vi "UHR-Fleezers Control (fpga) - 9.3.vi"() -> ()   [LabVIEW 2009]
doc: "UHR-Fleezers Instrument Control Code (fpga)"
uses:
  <vilib>/Platform/TimedLoop/XDataNode/XDataNode.xnode
  <vilib>/Platform/TimedLoop/XDataNode/loadlvalarms.vi
  <vilib>/Platform/TimedLoop/XDataNode/timing_clust.ctl
  <vilib>/Platform/TimedLoop/XDataNode/nitl_modes.ctl
  <vilib>/Platform/TimedLoop/XDataNode/wakeup.ctl
  <vilib>/eio/EIONode/EIONode.xnode
  <vilib>/rvi/eio/nirviEIOImplementation/nirviEIOImplementation.xnode
  <vilib>/rvi/eio/common/nirviEmuTemplateMethod_noerrors.vi
  <vilib>/rvi/eio/common/nirviEmuClasses.ctl
  <vilib>/eio/EIOMethodNode/EIOMethodNode.xnode
  <vilib>/rvi/eio/nirviEIOMethodImplementation/nirviEIOMethodImplementation.xnode
  <vilib>/rvi/DataTransferAndStorage/Container/XNode/niFpgaContainer.xnode
  <vilib>/rvi/interface/RandomDataEmulation/niFpgaRandomDataHandleErrors.vi
  <vilib>/rvi/interface/RandomDataEmulation/nirviRandomDataFPGAFIFO.vi
  <vilib>/rvi/DataTransferAndStorage/Container/Common/niFpgaContainerMethod.ctl
  <vilib>/rvi/DataTransferAndStorage/Container/Common/niFpgaTransferTypeControl.ctl
  <vilib>/Platform/TimedLoop/XDataNode/XDNodeRunTimeDep.lvlib
panel:
  in  "Tab Control":T1(tab)=enum."APD Counting"
  in  "AI Averages":u16=1 min=1 step=1
  in  "AI1 Sets to FIFO":T2={"Set 1"=TRUE, "Set 2"=TRUE, "Set 3"=FALSE}
  in  "N of AI1 Int Acq Sets":i16=2 min=1 max=3 step=1
  out "Number of AI channels":i16
  out "AI Late Counter":u32
  in  "ai count":u32=400
  out "AI late?":bool
  in  "+ phase":bool
  in  "Phase count adjustment":i16
  out "Relative phase":i16
  in  "DMA buffer timeout":i32
  in  "AI to FIFO":bool
  in  "Tab Control 2":T3(tab)
  in  "Swap F1 and F2":bool
  in  "Freq or Amp switch first":bool=TRUE
  in  "Cont. Scan":bool
  in  "Abort scan":bool
  in  "Cycles per step":u64
  in  "Scan BD":bool
  in  "Number of scans":u16
  in  "Scan steps":u64
  in  "Scan freq.  increment":i64
  out "Scanning":bool
  in  "Start scan":bool
  in  "OSK Bd 1":bool
  in  "Reset Bd 1":bool
  in  "RD":bool
  in  "PMODE":bool
  in  "OSK Bd 2":bool
  in  "Reset Bd 2":bool
  in  "Direct RF Box \nCommunication":bool
  in  "Data BD 2":u8 format="%08b"
  in  "Data BD 1":u8 format="%08b"
  in  "Address":u8 format="%02x"
  in  "Update Data":bool
  in  "FPGA Controls\n RF Box":bool
  in  "Number Interlace Cycles":u8=2 min=1 max=3
  in  "Interlace Off Parameters":u8=1 min=1 max=3
  in  "Interlace ON/OFF":bool
  out "DIO Relative phase":i16
  in  "Phase count adjustment (DIO)":i16
  in  "+ phase (DIO)":bool
  out "DIO Late Counter":u32
  out "DIO Late?":bool
  in  "DIO count 1 (ticks)":u32=400
  in  "DIO count 2 (ticks)":u32=400
  in  "DIO count 3 (ticks)":u32=400
  out "AI2 Y Sum Set 2":i16
  out "AI2 Y Sum Set 1":i16
  in  "FB Gains Set 1":T4={"proportional gain (Kc)"=10, "integral gain (Kc*Ts/Ti)"=5, "derivative gain (Kc*Td/Ts)"=0}
  in  "FB Setpoint Set 1":i16 min=0 step=1
  in  "FB Reset Set 1":bool
  in  "FB On/Off Set 1":bool
  in  "FB Reset Set 2":bool
  in  "FB On/Off Set 2":bool
  in  "FB Setpoint Set 2":i16 min=0 step=1
  in  "FB Gains Set 2":T4={"proportional gain (Kc)"=10, "integral gain (Kc*Ts/Ti)"=5, "derivative gain (Kc*Td/Ts)"=0}
  in  "FB output range 2":cluster{"output high":i16, "output low":i16}={"output high"=3000, "output low"=0}
  in  "FB output range 1":cluster{"output high":i16, "output low":i16}={"output high"=3000, "output low"=0}
  out "Scan I":u64
  in  "Amp switch delay":u16=5
  in  "Freq switch delay":u16
  in  "BD 2 Amplitude 1":u16
  in  "BD 1 Amplitude 1":u16
  in  "BD 2 Frequency 1":u64
  in  "BD 1 Frequency 1":u64
  in  "BD 2 Amplitude 2":u16
  in  "BD 1 Amplitude 2":u16
  in  "BD 2 Frequency 2":u64
  in  "BD 1 Frequency 2":u64
  in  "BD 2 Amplitude 3":u16
  in  "BD 1 Amplitude 3":u16
  in  "BD 2 Frequency 3":u64
  in  "BD 1 Frequency 3":u64
  out "Numeric":i32
  out "AO2 2":i16
  out "AO1 2":i16
  in  "1D or 2D Scan?":bool
  in  "Abort scan (MCL)":bool
  in  "MCL Scan Axis":bool
  in  "Cont. Scan (MCL)":bool
  out "Scan I (MCL)":u64
  in  "Number of scans (MCL)":u16
  out "Scanning MCL":bool
  in  "Scan steps (MCL)":u64
  in  "Cycles per step (MCL)":u64
  in  "Scan freq.  increment (MCL)":i16
  in  "Start scan (MCL)":bool
  in  "AO2":i16
  in  "AO1":i16
  out "MCL Late Counter":u32
  out "MCL Late?":bool
  in  "MCL count":u32=800
  out "MCL Relative Phase":i16
  in  "Phase count adjustment (MCL)":i16
  in  "+ phase (MCL)":bool
  in  "APD2 Trigger on Edge?":bool=TRUE
  in  "APD1 Trigger on Edge?":bool=TRUE
  in  "APD Gate Operating Mode":u8 max=2 step=1
  in  "Invert APD Gate":bool
  in  "APD Gate OFF Count":u32=100
  in  "APD Gate ON Count":u32=300
  out "APD Gate Late Counter":u32
  out "APD Gate Late?":bool
  out "APD Gate Relative Phase":i16
  in  "Phase count adjustment (APD Gate)":i16
  in  "+ phase (APD Gate)":bool
  out "APD 2 Counts 0":u32
  out "APD 2 Counts 1":u32
  out "APD 1 Counts 0":u32
  out "APD 1 Counts 1":u32
  out "APD out state":bool
  in  "APD 2 AO offset":i16
  in  "APD 1 AO offset":i16
  in  "APD 2 AO scale factor":i16=1
  in  "APD 1 AO scale factor":i16=1
  in  "APD to FIFO":bool
  in  "APD Acq Rate Count":u32=20000000
  out "APD Acq Late Counter":u32
  out "APD Acq Late?":bool
  out "APD Acq Relative Phase":i16
  in  "Phase Count Adjustment (APD Acq)":i16
  in  "+ phase (APD Acq)":bool
  in  "Green Filter Flipper":bool
  out "Green FB Signals":T5
  in  "Green FB Count":u32=1200
  out "Green Late Counter":u32
  out "Green FB Late?":bool
  out "Green FB Relative Phase":i16
  in  "Phase count adjustment (Green FB)":i16=10
  in  "+ phase (Green FB)":bool
  out "Green FB Sum":i16
  in  "Green int current ON count adj":u32=150
  in  "Current Out":u16=30000
  in  "Green FB On/Off":bool
  in  "Green FB Setpoint":i16=250 min=0 step=1
  in  "Green FB Gains":T4={"proportional gain (Kc)"=10, "integral gain (Kc*Ts/Ti)"=5, "derivative gain (Kc*Td/Ts)"=0}
  in  "Green FB Reset":bool
  in  "Operating Mode 2":u8=2 max=2 step=1
  in  "Invert GI 2":bool
  in  "Green interlace OFF count 2":u32=900
  in  "Green interlace ON count 2":u32=300
  out "GI Late Counter 2":u32
  out "GI Late? 2":bool
  out "GI Relative phase 2":i16
  in  "Phase count adjustment (GI) 2":i16=20
  in  "+ phase (GI) 2":bool
  in  "Green interlace OFF count":u32=100
  out "GI Relative phase":i16
  in  "Phase count adjustment (GI)":i16
  in  "+ phase (GI)":bool
  out "GI Late?":bool
  in  "Green interlace ON count":u32=300
  out "GI Late Counter":u32
  in  "Invert GI":bool
  in  "Operating Mode":u8 max=2 step=1
  in  "Connector0/DIO9":bool
  in  "Connector1/DIO32":bool
  in  "Connector1/DIO33":bool
  in  "Connector1/DIO34":bool
  in  "Chassis2/Mod4/AO1":u16
  in  "Extra DO Counts":u32=40000
  # "Only one of these can be on\nat a time:"
  # "Raster Scan AOD"
  # "1 (X)"
  # "2 (Y)"
  # "IR Intensity Feedback (RF BD 1)"
  # "AO1 (Y)"
  # "2D"
  # "1D"
  # "AO2 (X)"
  # "APD AO for aligning"
  # "Detection Loop"
  # "Green fluorescent laser digital gate interlacing loop"
  # "0 Forced ON\n1 Forced OFF\n2 Interlacing"
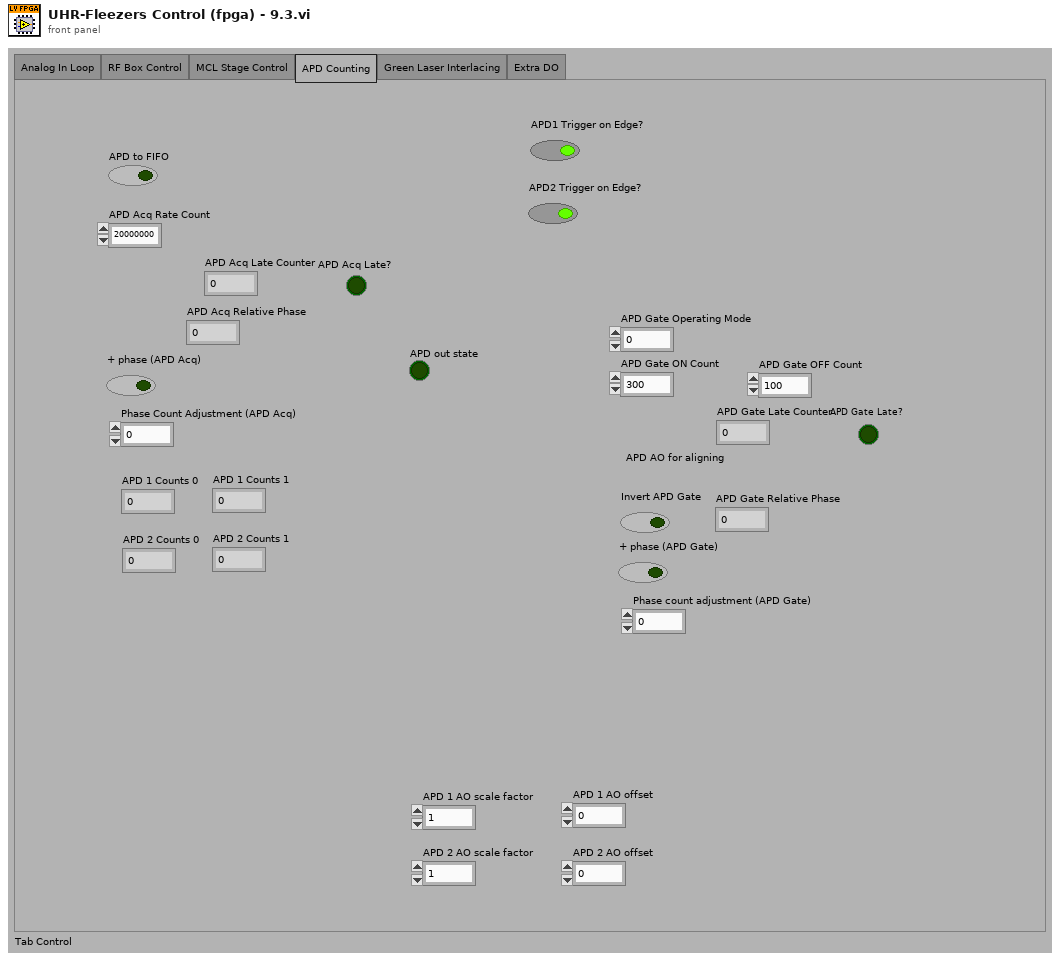
[diagram p1: front panel]
types:
  T1 = enum32{"Analog In Loop", "RF Box Control", "MCL Stage Control", "APD Counting", "Green Laser Interlacing", "Extra DO"}
  T2 = cluster{"Set 1":bool, "Set 2":bool, "Set 3":bool}
  T3 = enum32{"Controls", "Interlacing Frequency and Amplitude Values"}
  T4 = cluster{"proportional gain (Kc)":i16, "integral gain (Kc*Ts/Ti)":i16, "derivative gain (Kc*Td/Ts)":i16}
  T5 = cluster{"Green FB Ch 0":i16, "Green FB Ch 1":i16, "Green FB Ch 2":i16}
  T6 = typedef "nirviEmuClasses.ctl" = enum16{"IO Read", "IO Write", "Method", "Property Read", "Property Write"}
  T7 = typedef "XDNodeRunTimeDep.lvlib/timing_clust.ctl" = cluster{"Expected End [f-1]":u64, "Actual End [f-1]":u64, "Finished Late? [f-1]":bool, "Expected End [i-1]":u64, "Actual End [i-1]":u64, "Finished Late? [i-1]":bool, "Expected Start [i]":u64, "Actual Start [i]":u64, "Expected Start [f]":u64, "Actual Start [f]":u64, "Source Name":string, "Structure Name":string, "Period":i64, "Deadline":i64, "Offset":i64, "Start":i64, "Priority":i32, "Timeout":i32, "Mode":T8, "Wakeup Reason":T9, "Error":errorcluster, "Source Type":string, "Secondary Source Type":string, "Global End Time":u64, "Global Start Time":u64, "Frame Duration":u64, "Iteration Duration":u64, "Assigned CPU":i32, "I/O Scan Engine Mode":u32}
  T8 = typedef "XDNodeRunTimeDep.lvlib/nitl_modes.ctl" = enum32{"No Change", "Process missed periods, maintain original phase", "Discard missed periods, maintain original phase", "Process missed periods, ignore original phase", "Discard missed periods, ignore original phase"}
  T9 = typedef "XDNodeRunTimeDep.lvlib/wakeup.ctl" = enum32{"Normal", "Aborted", "Asynchronous wakeup", "Timing source error", "Timed loop error", "Timeout"}
  T10 = typedef "niFpgaContainerMethod.ctl" = enum16{"Write", "Read", "Clear", "Get Number of Elements to Write", "Get Number of Elements to Read", "Enable", "Disable", "Flush and Disable", "Get Stream State"}
  T11 = typedef "niFpgaTransferTypeControl.ctl" = enum16{"Target-Scoped", "Host to Target - DMA", "Target to Host - DMA", "Peer to Peer Reader", "Peer to Peer Writer", "Bidirectional"}
  T12 = cluster{"Chassis2/Mod1/AI0":i16, "Chassis2/Mod1/AI1":i16, "Chassis2/Mod1/AI2":i16}
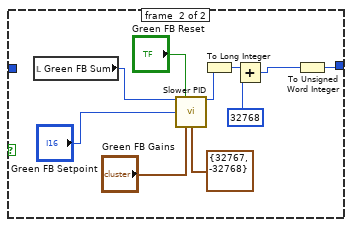
[diagram p2: hidden frame]
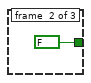
[diagram p3: hidden frame]
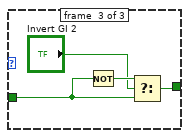
[diagram p4: hidden frame]
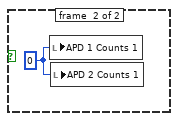
[diagram p5: hidden frame]
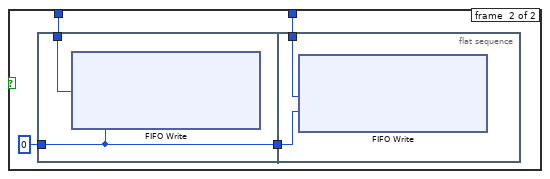
[diagram p6: hidden frame]
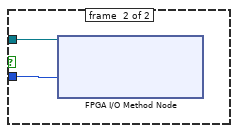
[diagram p7: hidden frame]
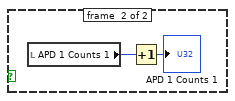
[diagram p8: hidden frame]
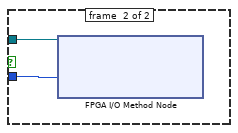
[diagram p9: hidden frame]
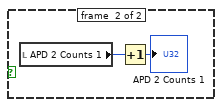
[diagram p10: hidden frame]
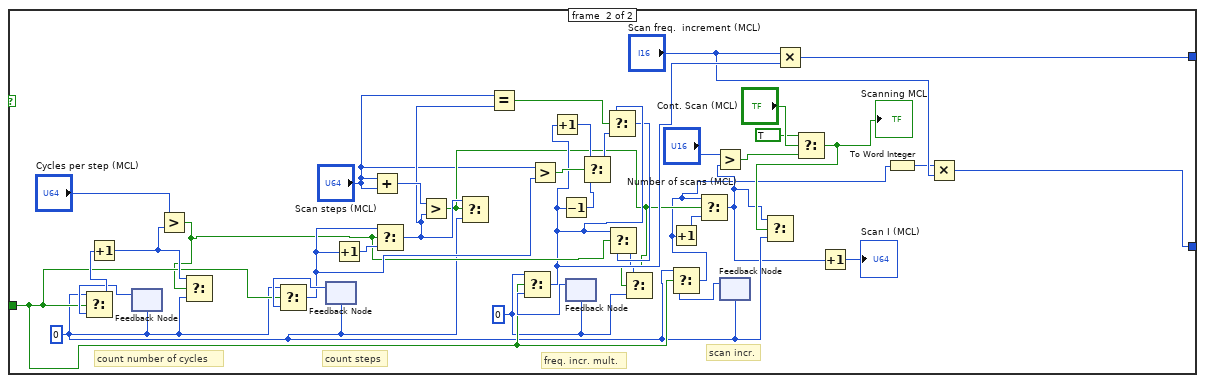
[diagram p11: hidden frame]
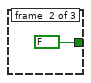
[diagram p12: hidden frame]
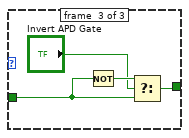
[diagram p13: hidden frame]
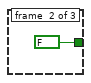
[diagram p14: hidden frame]
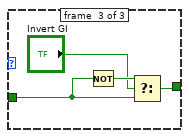
[diagram p15: hidden frame]
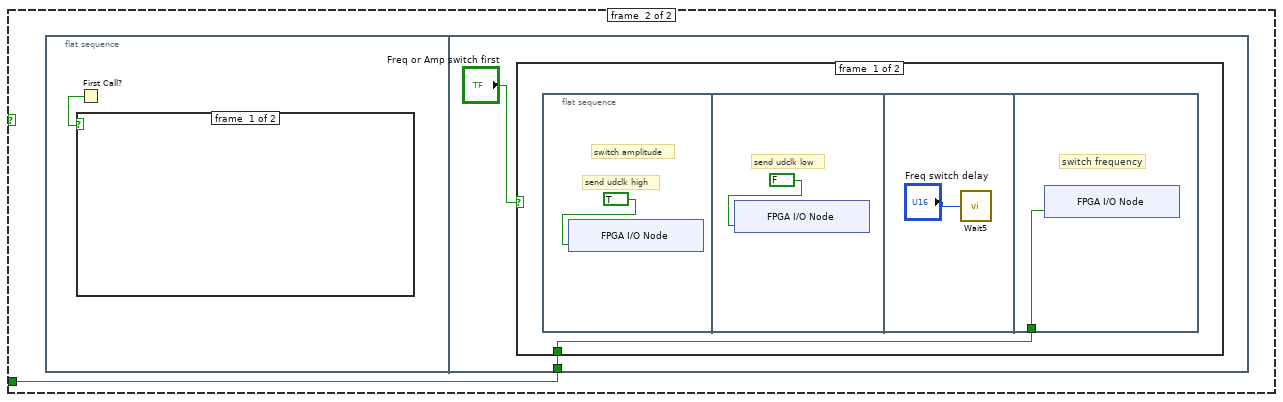
[diagram p16: hidden frame]
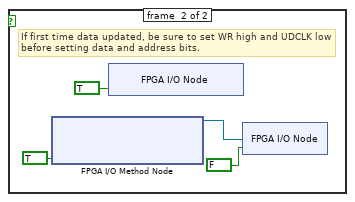
[diagram p17: hidden frame]
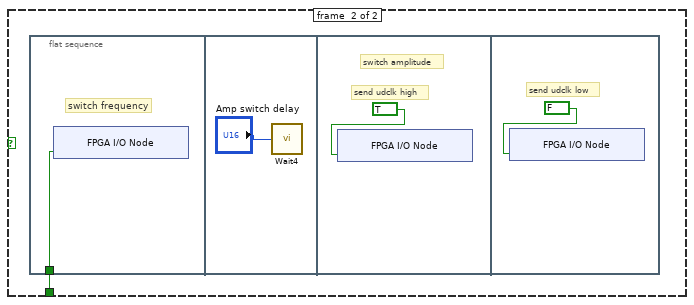
[diagram p18: hidden frame]
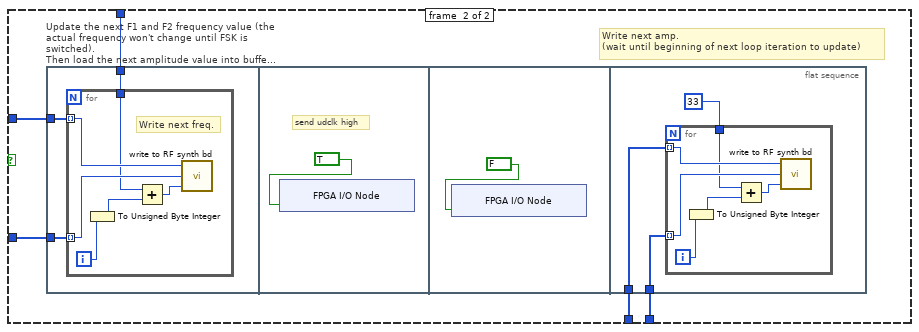
[diagram p19: hidden frame]
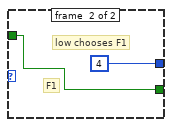
[diagram p20: hidden frame]
diagram:
  # "timing array current index"
  # "timing array"
  # "timing counter (phase adjusted here)"
  # "late counter"
  n1 = flat-sequence "FPGA initialization to do before running any of the loops" {
    tunnel: [u32 0 ("DIO count 3 (ticks)")] -> w1
    tunnel: [w10] -> _
    frame #0 {
      # "This is a kludge to let host programs know how many channels of data are in the DMA stream.  Set by hand."
      # "Start up expansion chassis early\nto avoid delays later"
      # "This pin controls udclk on the RF boards.\nWhen initially configuring the boards, this pin needs to be\nconfigured as a high impedance input.  Later it will be switched\nto an output."
      # "Initial setting of DIO data and \naddress to low (before reset).  \nThis needs to happen before the other\ncontrol method loops execute."
      n2 = xnode "FPGA I/O Node"("Chassis2/Mod4/AO0"=u16 0) -> ("Chassis2/Mod1/AI0"=w10:i16)  [unwired: 2 in, 2 out]
      n3 = xnode "FPGA I/O Method Node"("Enable"=FALSE) -> ()  [unwired: 1 in, 1 out]
      n4 = xnode "FPGA I/O Node"("Connector1/DIO0"=FALSE, "Connector1/DIO1"=FALSE, "Connector1/DIO2"=FALSE, "Connector1/DIO3"=FALSE, "Connector1/DIO4"=FALSE, "Connector1/DIO5"=FALSE, "Connector1/DIO6"=FALSE, "Connector1/DIO7"=FALSE, "Connector1/DIO8"=FALSE, "Connector1/DIO9"=FALSE, "Connector1/DIO10"=FALSE, "Connector1/DIO11"=FALSE, "Connector1/DIO12"=FALSE, "Connector1/DIO13"=FALSE, "Connector1/DIO15"=FALSE, "Connector1/DIO20"=FALSE, "Connector1/DIO21"=FALSE, "Connector1/DIO22"=FALSE, "Connector1/DIO23"=FALSE, "Connector1/DIO24"=FALSE, "Connector1/DIO25"=FALSE, "Connector1/DIO26"=FALSE, "Connector1/DIO27"=FALSE, "Connector1/DIO14"=FALSE) -> ()  [unwired: 24 in, 24 out]
      "Number of AI channels" <- i16 12 ("Number of AI channels")
    }
  }
  n5 = local read "AO1"() -> (w5:i16)
  n6 = local read "AO2"() -> (w4:i16)
  n7 = node-c288() -> (w3:T7)  [unwired: 1 in]
  n8 = while "APD 1 Counter" {
    tunnel: w1 -> [_]
    stop <- FALSE stop-if-true
    n9 = flat-sequence {
      frame #0 {
        n10 = case shown="False" "APD1 Trigger on Edge?" {
          tunnel: refnum<k21> "Connector0/DIO0" ("APD 1 DO") -> [w398 w423]
          tunnel: -1 ("Timeout") -> [w397 w422]
          frame #0 {
            n11 = xnode "FPGA I/O Method Node"("FPGA I/O In"=w398, "Timeout"=w397) -> ()  [unwired: 2 out]
          }
          frame #1 {
            n12 = xnode "FPGA I/O Method Node"("FPGA I/O In"=w423, "Timeout"=w422) -> ()  [unwired: 2 out]
          }
        }
      }
      frame #1 {
        n13 = local read "APD out state"() -> (w447:bool)
        n14 = case shown="False" w447 {
          frame #0 {
            n15 = local read "APD 1 Counts 0"() -> (w449:u32)
            n16 = Increment(x=w449) -> (x+1=→"APD 1 Counts 0":u32)
          }
          frame #1 {
            n17 = local read "APD 1 Counts 1"() -> (w451:u32)
            n18 = Increment(x=w451) -> (x+1=→"APD 1 Counts 1":u32)
          }
        }
      }
    }
  }
  n19 = while "APD 2 Counter" {
    tunnel: w1 -> [_]
    stop <- FALSE stop-if-true
    n20 = flat-sequence {
      frame #0 {
        n21 = case shown="False" "APD2 Trigger on Edge?" {
          tunnel: refnum<k21> "Connector0/DIO1" ("APD 2 DO") -> [w457 w482]
          tunnel: -1 ("Timeout") -> [w456 w481]
          frame #0 {
            n22 = xnode "FPGA I/O Method Node"("FPGA I/O In"=w457, "Timeout"=w456) -> ()  [unwired: 2 out]
          }
          frame #1 {
            n23 = xnode "FPGA I/O Method Node"("FPGA I/O In"=w482, "Timeout"=w481) -> ()  [unwired: 2 out]
          }
        }
      }
      frame #1 {
        n24 = local read "APD out state"() -> (w506:bool)
        n25 = case shown="False" w506 {
          frame #0 {
            n26 = local read "APD 2 Counts 0"() -> (w508:u32)
            n27 = Increment(x=w508) -> (x+1=→"APD 2 Counts 0":u32)
          }
          frame #1 {
            n28 = local read "APD 2 Counts 1"() -> (w510:u32)
            n29 = Increment(x=w510) -> (x+1=→"APD 2 Counts 1":u32)
          }
        }
      }
    }
  }
  n30 = while "DAQ AI set 1" {
    shift-right: [w511] -> _
    shift-left: w1 -> [w516]
    stop <- FALSE stop-if-true
    n31 = flat-sequence {
      tunnel: w516 -> [w526]
      tunnel: [w527] -> w514
      tunnel: [w526] -> w513
      tunnel: [w537] -> w524
      tunnel: [w536] -> w523
      tunnel: [w535] -> w522
      tunnel: [w534] -> w521
      tunnel: [w533] -> w520
      tunnel: [w532] -> w519
      tunnel: [w531] -> w518
      tunnel: [w530] -> w517
      tunnel: [w529] -> w515
      tunnel: w514 -> [w529]
      tunnel: w513 -> [w528]
      tunnel: [w528] -> w512
      tunnel: [w714] -> w511
      tunnel: w524 -> [w752]
      tunnel: w523 -> [w751]
      tunnel: w522 -> [w735]
      tunnel: w521 -> [w750]
      tunnel: w520 -> [w739]
      tunnel: w519 -> [w738]
      tunnel: w518 -> [w737]
      tunnel: w517 -> [w736]
      tunnel: w515 -> [w731]
      tunnel: w512 -> [w728]
      frame #0 {
        n32 = call "Loop Timer3"("Count(Ticks)"=w526) -> ("Tick Count(Ticks)"=w527:u32)
      }
      frame #1 {
        n33 = xnode "FPGA I/O Node"("Connector1/DIO31"=TRUE ("Connector1/DIO33")) -> ("Connector0/AI0"=w537:i16, "Connector0/AI1"=w536:i16, "Connector0/AI2"=w535:i16, "Connector0/AI3"=w534:i16, "Connector0/AI4"=w533:i16, "Connector0/AI5"=w532:i16, "Connector0/AI6"=w531:i16, "Connector0/AI7"=w530:i16)  [unwired: 9 in, 9 out]
      }
      frame #2 {
        # "Adjust phase after data acquired if button pressed"
        n34 = feedback #1(i16 1) -> (w743:i16)
        n35 = Increment(x=w743) -> (x+1=w749:i16)
        n36 = Greater?(x=w749, y="N of AI1 Int Acq Sets") -> (0:w746:bool)
        n37 = Select(t=i16 1, s=w746, f=w749) -> (s? t:f=w748:i16)
        n38 = feedback #2(FALSE ("AI to FIFO")) -> (w733:bool)
        n39 = case shown="1, Default" w743 {
          tunnel: w735 -> [w755 w759 _]
          tunnel: "AI1 Sets to FIFO" -> [w757 w761 w764]
          tunnel: [w756 w760 w763] -> w740
          tunnel: ["AI to FIFO" w758 w762] -> w732
          tunnel: w733 -> [_ w758 w762]
          frame #0 {
            n40 = Unbundle By Name(w757) -> ("Set 1"=w756:bool)
            "AI2 Y Sum Set 1" <- w755
          }
          frame #1 {
            n41 = Unbundle By Name(w761) -> ("Set 2"=w760:bool)
            "AI2 Y Sum Set 2" <- w759
          }
          frame #2 {
            n42 = Unbundle By Name(w764) -> ("Set 3"=w763:bool)
          }
        }
        n43 = And(x=w740, y=w732) -> (x .and. y?=w742:bool)
        n44 = case shown="True" w742 {
          tunnel: w752 -> [_ w769]
          tunnel: w751 -> [_ w770]
          tunnel: w735 -> [_ w771]
          tunnel: w750 -> [_ w772]
          tunnel: w739 -> [_ w776]
          tunnel: w738 -> [_ w775]
          tunnel: w737 -> [_ w774]
          tunnel: w736 -> [_ w773]
          frame #0 {
          }
          frame #1 {
            n45 = Greater?(x="AI Averages", y=u16 1) -> (0:w767:bool)
            n46 = case shown="True" w767 {
              tunnel: w776 -> [w787 w844]
              tunnel: w775 -> [w786 w843]
              tunnel: w774 -> [w785 w842]
              tunnel: w773 -> [w784 w841]
              tunnel: w772 -> [w783 w840]
              tunnel: w771 -> [w788 w839]
              tunnel: w770 -> [w789 w838]
              tunnel: w769 -> [w790 w837]
              tunnel: "AI Averages" -> [_ w824]
              tunnel: "DMA buffer timeout" -> [w778 w821]
              frame #0 {
                n47 = Join Numbers(hi=w790, lo=w789) -> ((hi.lo)=w782:u32)
                n48 = Join Numbers(hi=w788, lo=w783) -> ((hi.lo)=w781:u32)
                n49 = Join Numbers(hi=w787, lo=w786) -> ((hi.lo)=w780:u32)
                n50 = Join Numbers(hi=w785, lo=w784) -> ((hi.lo)=w779:u32)
                n51 = Build Array(w782, w781, w780, w779) -> (w777:u32[])
                n52 = for {
                  tunnel: w777 -> [w792] mode=indexing
                  tunnel: w778 -> [w793]
                  n53 = To Unsigned Long Integer(number=w792) -> (unsigned 32bit integer=w791:u32)
                  n54 = xnode ("FIFO Write")("Element"=w791, "Timeout"=w793) -> ()  [unwired: 1 in, 2 out]
                }
              }
              frame #1 {
                w828 = u16 0
                n55 = To Long Integer(number=w837) -> (32bit integer=w830:i32)
                n56 = To Long Integer(number=w838) -> (32bit integer=w847:i32)
                n57 = To Long Integer(number=w839) -> (32bit integer=w846:i32)
                n58 = To Long Integer(number=w840) -> (32bit integer=w845:i32)
                n59 = To Long Integer(number=w844) -> (32bit integer=w836:i32)
                n60 = To Long Integer(number=w843) -> (32bit integer=w835:i32)
                n61 = To Long Integer(number=w842) -> (32bit integer=w834:i32)
                n62 = To Long Integer(number=w841) -> (32bit integer=w833:i32)
                n63 = Build Array(w830, w847, w846, w845, w836, w835, w834, w833) -> (w819:i32[])
                n64 = feedback #3(w819) -> (w832:i32[])
                n65 = Add(x=w819, y=w832) -> (x+y=w831:i32[])
                n66 = feedback #4(w828) -> (w826:u16)
                n67 = Increment(x=w826) -> (x+1=w823:u16)
                n68 = Equal?(x=w823, y=u16 1) -> (x = y?=w822:bool)
                n69 = Select(t=w819, s=w822, f=w831) -> (s? t:f=w820:i32[])
                n70 = Greater Or Equal?(x=w823, y=w824) -> (x >= y?=w825:bool)
                n71 = Select(t=w828, s=w825, f=w823) -> (s? t:f=w827:u16)
                n72 = case shown="True" w825 {
                  tunnel: w820 -> [_ w849]
                  tunnel: w821 -> [_ w848]
                  frame #0 {
                  }
                  frame #1 {
                    n73 = for {
                      tunnel: w849 -> [w851] mode=indexing
                      tunnel: w848 -> [w852]
                      n74 = To Unsigned Long Integer(number=w851) -> (unsigned 32bit integer=w850:u32)
                      n75 = xnode ("FIFO Write")("Element"=w850, "Timeout"=w852) -> ()  [unwired: 1 in, 2 out]
                    }
                  }
                }
              }
            }
          }
        }
        n76 = feedback #5(w731) -> (w730:u32)
        n77 = Subtract(x=w731, y=w730) -> (x-y=w729:u32)
        n78 = Subtract(x=w729, y=w728) -> (x-y=w725:u32)
        n79 = Subtract(x="ai count", y=w725) -> (x-y=w715:u32)
        n80 = Greater?(x=w725, y=u32 0) -> (0:w723:bool)
        "AI late?" <- w723
        n81 = feedback #6(u32 0) -> (w721:u32)
        n82 = Increment(x=w721) -> (x+1=w720:u32)
        n83 = Select(t=w720, s=w723, f=w721) -> (s? t:f=w722:u32)
        "AI Late Counter" <- w722
        n84 = xnode "I/O Node"("Connector1/DIO31"=FALSE ("Connector1/DIO34")) -> ()  [unwired: 1 in, 1 out]
        n85 = Boolean To (0,1)(Boolean="+ phase") -> (0, 1=w717:i16)
        n86 = Multiply(x=w717, y="Phase count adjustment") -> (x*y=w711:i16)
        n87 = feedback #7(i16 0) -> (w713:i16)
        n88 = Add(x=w715, y=w711) -> (x+y=w714:u32)
        n89 = Subtract(x=w713, y=w711) -> (x-y=w712:i16)
        "Relative phase" <- w712
      }
    }
  }
  n90 = while "RF box board DIO control: parallel communication" {
    shift-right: [w897] -> _
    shift-left: w1 -> [w896]
    shift-right: [w895] -> _
    shift-left: FALSE ("Swap F1 and F2") -> [w894]
    stop <- FALSE stop-if-true
    n91 = flat-sequence {
      tunnel: w894 -> [w901]
      tunnel: w896 -> [w899]
      tunnel: [w901] -> w893
      tunnel: [w900] -> w892
      tunnel: [w899] -> w891
      tunnel: [w907] -> w897
      tunnel: [w906] -> w895
      tunnel: w893 -> [w905]
      tunnel: w892 -> [w903]
      tunnel: w891 -> [w902]
      frame #0 {
        n92 = call "Loop Timer"("Count(Ticks)"=w899) -> ("Tick Count(Ticks)"=w900:u32)
      }
      frame #1 {
        n93 = flat-sequence {
          tunnel: ["FPGA Controls\n RF Box"] -> w904
          tunnel: w905 -> [w908]
          tunnel: [w1057] -> w907
          tunnel: [w1077] -> w906
          tunnel: w904 -> [w1076]
          tunnel: w903 -> [w1070]
          tunnel: w902 -> [w1067]
          frame #0 {
            n94 = case shown="True" "FPGA Controls\n RF Box" {
              tunnel: w908 -> [_ w910]
              frame #0 {
              }
              frame #1 {
                n95 = flat-sequence {
                  tunnel: w910 -> [w955]
                  frame #0 {
                    n96 = First Call?() -> (First Call?: T/F=w911:bool)
                    n97 = case shown="True" w911 {
                      frame #0 {
                      }
                      frame #1 {
                        # "If first time data updated, be sure to set WR high and UDCLK low\nbefore setting data and address bits."
                        n98 = xnode "FPGA I/O Method Node"("Enable"=TRUE) -> ("FPGA I/O Out"=w913:refnum<k21>)  [unwired: 1 in]
                        n99 = xnode "FPGA I/O Node"("Connector1/DIO15"=TRUE) -> ()  [unwired: 1 in, 1 out]
                        n100 = xnode "FPGA I/O Node"("I/O Item"=FALSE ("Connector1/DIO30"), "FPGA I/O In"=w913) -> ()  [unwired: 1 out]
                      }
                    }
                  }
                  frame #1 {
                    n101 = case shown="True" "Freq or Amp switch first" {
                      tunnel: w955 -> [w957 w1001]
                      frame #0 {
                        n102 = flat-sequence {
                          tunnel: w957 -> [w987]
                          frame #0 {
                            # "switch amplitude"
                            # "send udclk high"
                            n103 = xnode "FPGA I/O Node"("Connector1/DIO30"=TRUE ("Connector1/DIO15")) -> ()  [unwired: 1 in, 1 out]
                          }
                          frame #1 {
                            # "send udclk low"
                            n104 = xnode "FPGA I/O Node"("Connector1/DIO30"=FALSE ("Connector1/DIO15")) -> ()  [unwired: 1 in, 1 out]
                          }
                          frame #2 {
                            n105 = call "Wait5"("Count(Ticks)"="Freq switch delay") -> ()  [unwired: 1 out]
                          }
                          frame #3 {
                            # "switch frequency"
                            n106 = xnode "FPGA I/O Node"("Connector1/DIO36"=w987) -> ()  [unwired: 1 in, 1 out]
                          }
                        }
                      }
                      frame #1 {
                        n107 = flat-sequence {
                          tunnel: w1001 -> [w1002]
                          frame #0 {
                            # "switch frequency"
                            n108 = xnode "FPGA I/O Node"("Connector1/DIO36"=w1002) -> ()  [unwired: 1 in, 1 out]
                          }
                          frame #1 {
                            n109 = call "Wait4"("Count(Ticks)"="Amp switch delay") -> ()  [unwired: 1 out]
                          }
                          frame #2 {
                            # "switch amplitude"
                            # "send udclk high"
                            n110 = xnode "FPGA I/O Node"("Connector1/DIO30"=TRUE ("Connector1/DIO15")) -> ()  [unwired: 1 in, 1 out]
                          }
                          frame #3 {
                            # "send udclk low"
                            n111 = xnode "FPGA I/O Node"("Connector1/DIO30"=FALSE ("Connector1/DIO15")) -> ()  [unwired: 1 in, 1 out]
                          }
                        }
                      }
                    }
                  }
                }
              }
            }
          }
          frame #1 {
            # "This is the prior cycle's on time"
            # "increment timing\nindex, reset to 0 if \nend of matrix"
            # "Reset to begginning (1) when number of cycles reached."
            # "timing index"
            # "build byte stacks for writing data\n(must correspond to addresses array constant)"
            # "Timing housekeeping"
            # "Adjust phase if late\n(maintains constant phase relationship between cycles)"
            n112 = feedback #8(u8 0 ("t")) -> (w1073:u8)
            n113 = Increment(x=w1073) -> (x+1=w1117:u8)
            n114 = Increment(x="Number Interlace Cycles") -> (x+1=w1112:u8)
            n115 = Equal?(x=w1117, y=w1112) -> (x = y?=w1119:bool)
            n116 = Select(t=u8 1, s=w1119, f=w1117) -> (s? t:f=w1072:u8)
            n117 = Increment(x=w1072) -> (x+1=w1114:u8)
            n118 = Equal?(x=w1114, y=w1112) -> (x = y?=w1115:bool)
            n119 = Select(t=u8 1, s=w1115, f=w1114) -> (s? t:f=w1111:u8)
            n120 = Select(t=w1111, s="Interlace ON/OFF", f="Interlace Off Parameters") -> (s? t:f=w1095:u8)
            n121 = case shown="1, Default" w1095 {
              tunnel: [w1191 "BD 1 Frequency 2" "BD 1 Frequency 3"] -> w1107
              tunnel: [w1190 "BD 2 Frequency 2" "BD 2 Frequency 3"] -> w1096
              tunnel: ["BD 2 Amplitude 1" "BD 2 Amplitude 2" "BD 2 Amplitude 3"] -> w1045
              tunnel: [w1179 w1249 "BD 1 Amplitude 3"] -> w1048
              frame #0 {
                w1186 = u8 0 ("f")
                n122 = local read "Scanning"() -> (w1192:bool)
                n123 = Or(x=w1192, y="Start scan") -> (x .or. y?=w1184:bool)
                n124 = Not(x="Abort scan") -> (.not. x?=w1182:bool)
                n125 = And(x=w1182, y=w1184) -> (x .and. y?=w1181:bool)
                n126 = case "Raster scan" shown="True" w1181 {
                  tunnel: [i16 0 w1238] -> w1187
                  tunnel: "Start scan" -> [_ w1223]
                  frame #0 {
                    n127 = local write "Scanning"(FALSE ("scanning")) -> ()
                  }
                  frame #1 {
                    w1207 = i64 0
                    w1206 = u64 0
                    # "scan incr."
                    # "freq. incr. mult."
                    # "count steps"
                    # "count number of cycles"
                    n128 = feedback #9(w1206) -> (w1235:u64)
                    n129 = Select(t=w1206, s=w1223, f=w1235) -> (s? t:f=w1237:u64)
                    n130 = Increment(x=w1237) -> (x+1=w1234:u64)
                    n131 = Greater?(x="Cycles per step", y=w1234) -> (0:w1216:bool)
                    n132 = Select(t=w1234, s=w1216, f=w1206) -> (s? t:f=w1233:u64)
                    n133 = feedback #10(w1206) -> (w1232:u64)
                    n134 = Select(t=w1206, s=w1223, f=w1232) -> (s? t:f=w1227:u64)
                    n135 = Increment(x=w1227) -> (x+1=w1231:u64)
                    n136 = Add(x="Scan steps", y="Scan steps") -> (x+y=w1230:u64)
                    n137 = Select(t=w1227, s=w1216, f=w1231) -> (s? t:f=w1211:u64)
                    n138 = Greater?(x=w1230, y=w1211) -> (0:w1210:bool)
                    n139 = Select(t=w1211, s=w1210, f=w1206) -> (s? t:f=w1228:u64)
                    n140 = Equal?(x="Scan steps", y=w1211) -> (x = y?=w1215:bool)
                    n141 = Greater?(x="Scan steps", y=w1227) -> (0:w1226:bool)
                    n142 = feedback #11(w1207) -> (w1229:i64)
                    n143 = Select(t=w1207, s=w1223, f=w1229) -> (s? t:f=w1213:i64)
                    n144 = Increment(x=w1213) -> (x+1=w1225:i64)
                    n145 = Decrement(x=w1213) -> (x-1=w1224:i64)
                    n146 = Select(t=w1225, s=w1226, f=w1224) -> (s? t:f=w1214:i64)
                    n147 = Select(t=w1213, s=w1215, f=w1214) -> (s? t:f=w1212:i64)
                    n148 = Select(t=w1213, s=w1216, f=w1212) -> (s? t:f=w1208:i64)
                    n149 = Select(t=w1208, s=w1210, f=w1207) -> (s? t:f=w1209:i64)
                    n150 = feedback #12(w1206) -> (w1222:u64)
                    n151 = Select(t=w1206, s=w1223, f=w1222) -> (s? t:f=w1218:u64)
                    n152 = Increment(x=w1218) -> (x+1=w1219:u64)
                    n153 = Select(t=w1218, s=w1210, f=w1219) -> (s? t:f=w1217:u64)
                    n154 = Greater?(x="Number of scans", y=w1217) -> (0:w1203:bool)
                    n155 = Multiply(x="Scan freq.  increment", y=w1213) -> (x*y=w1238:i64)
                    n156 = Select(t=TRUE, s="Cont. Scan", f=w1203) -> (s? t:f=w1202:bool)
                    "Scanning" <- w1202
                    n157 = Select(t=w1217, s=w1202, f=w1206) -> (s? t:f=w1220:u64)
                    n158 = Increment(x=w1217) -> (x+1=→"Scan I":u64)
                  }
                }
                n159 = case shown="True" "FB On/Off Set 1" {
                  tunnel: "BD 1 Amplitude 1" -> [w1240 _]
                  tunnel: [w1240 w1241] -> w1179
                  frame #0 {
                  }
                  frame #1 {
                    n160 = local read "AI2 Y Sum Set 1"() -> (w1243:i16)
                    n161 = call "Slower PID.vi"("process variable"=w1243, "reset?"="FB Reset Set 1", "setpoint"="FB Setpoint Set 1", "PID gains (x 2^8)"="FB Gains Set 1", "output range"="FB output range 1") -> ("output"=w1246:i16)  [unwired: 10 out]
                    n162 = To Unsigned Word Integer(number=w1246) -> (unsigned 16bit integer=w1241:u16)
                  }
                }
                n163 = Select(t=w1186, s="Scan BD", f=w1187) -> (s? t:f=w1185:i64)
                n164 = Select(t=w1187, s="Scan BD", f=w1186) -> (s? t:f=w1188:i64)
                n165 = Add(x=w1185, y="BD 2 Frequency 1") -> (x+y=w1190:u64)
                n166 = Add(x="BD 1 Frequency 1", y=w1188) -> (x+y=w1191:u64)
              }
              frame #1 {
                n167 = case shown="True" "FB On/Off Set 2" {
                  tunnel: [w1254 w1255] -> w1249
                  tunnel: "BD 1 Amplitude 2" -> [w1254 _]
                  frame #0 {
                  }
                  frame #1 {
                    n168 = local read "AI2 Y Sum Set 2"() -> (w1260:i16)
                    n169 = call "Slower PID.vi"("process variable"=w1260, "reset?"="FB Reset Set 2", "setpoint"="FB Setpoint Set 2", "PID gains (x 2^8)"="FB Gains Set 2", "output range"="FB output range 2") -> ("output"=w1257:i16)  [unwired: 10 out]
                    n170 = To Unsigned Word Integer(number=w1257) -> (unsigned 16bit integer=w1255:u16)
                  }
                }
              }
              frame #2 {
              }
            }
            n171 = feedback #13(w1070) -> (w1069:u32)
            n172 = Subtract(x=w1070, y=w1069) -> (x-y=w1068:u32)
            n173 = Select(t=w1072, s="Interlace ON/OFF", f="Interlace Off Parameters") -> (s? t:f=w1110:u8)
            n174 = Subtract "The error"(x=w1068, y=w1067) -> (x-y=w1065:u32)
            n175 = case shown="3" w1110 {
              tunnel: ["DIO count 1 (ticks)" "DIO count 2 (ticks)" "DIO count 3 (ticks)"] -> w1066
              frame #0 {
              }
              frame #1 {
              }
              frame #2 {
              }
            }
            n176 = Greater?(x=w1065, y=u32 0) -> (0:w1060:bool)
            "DIO Late?" <- w1060
            n177 = feedback #14(u32 0) -> (w1062:u32)
            n178 = Increment(x=w1062) -> (x+1=w1061:u32)
            n179 = Select(t=w1061, s=w1060, f=w1062) -> (s? t:f=w1063:u32)
            "DIO Late Counter" <- w1063
            n180 = Subtract(x=w1066, y=w1065) -> (x-y=w1058:u32)
            n181 = Boolean To (0,1)(Boolean="+ phase (DIO)") -> (0, 1=w1055:i16)
            n182 = Multiply(x=w1055, y="Phase count adjustment (DIO)") -> (x*y=w1051:i16)
            n183 = feedback #15(i16 0) -> (w1053:i16)
            n184 = Subtract(x=w1053, y=w1051) -> (x-y=w1052:i16)
            "DIO Relative phase" <- w1052
            n185 = Split Number(x=w1096) -> (hi(x)=w1101:u32, lo(x)=w1100:u32)
            n186 = Split Number(x=w1107) -> (hi(x)=w1106:u32, lo(x)=w1105:u32)
            n187 = Split Number(x=w1101) -> (lo(x)=w1099:u16)  [unwired: 1 out]
            n188 = Split Number(x=w1100) -> (hi(x)=w1098:u16, lo(x)=w1097:u16)
            n189 = Split Number(x=w1106) -> (lo(x)=w1104:u16)  [unwired: 1 out]
            n190 = Split Number(x=w1105) -> (hi(x)=w1103:u16, lo(x)=w1102:u16)
            n191 = Split Number(x=w1048) -> (hi(x)=w1050:u8, lo(x)=w1049:u8)
            n192 = Split Number(x=w1099) -> (hi(x)=w1087:u8, lo(x)=w1086:u8)
            n193 = Split Number(x=w1098) -> (hi(x)=w1085:u8, lo(x)=w1084:u8)
            n194 = Split Number(x=w1097) -> (hi(x)=w1083:u8, lo(x)=w1082:u8)
            n195 = Split Number(x=w1045) -> (hi(x)=w1047:u8, lo(x)=w1046:u8)
            n196 = Add(x=w1058, y=w1051) -> (x+y=w1057:u32)
            n197 = Split Number(x=w1104) -> (hi(x)=w1094:u8, lo(x)=w1093:u8)
            n198 = Split Number(x=w1103) -> (hi(x)=w1092:u8, lo(x)=w1091:u8)
            n199 = Split Number(x=w1102) -> (hi(x)=w1090:u8, lo(x)=w1089:u8)
            n200 = Build Array "BD 1 A Stack"(w1050, w1049) -> (w1079:u8[])
            n201 = Build Array "BD 2 nu Stack"(w1087, w1086, w1085, w1084, w1083, w1082) -> (w1081:u8[])
            n202 = Build Array "BD 2 A Stack"(w1047, w1046) -> (w1078:u8[])
            n203 = Build Array "BD 1 nu Stack"(w1094, w1093, w1092, w1091, w1090, w1089) -> (w1088:u8[])
            n204 = case shown="2" w1095 {
              tunnel: [w1171 w1174] -> w1077
              tunnel: [u8 10 u8 4] -> w1080
              tunnel: "Swap F1 and F2" -> [w1172 w1174]
              frame #0 {
                # "F2"
                n205 = Not(x=w1172) -> (.not. x?=w1171:bool)
              }
              frame #1 {
                # "low chooses F1"
                # "F1"
              }
            }
            n206 = case "If FPGA is controlling (toggling) RF synth" shown="True" w1076 {
              tunnel: w1088 -> [_ w1124]
              tunnel: w1081 -> [_ w1123]
              tunnel: w1080 -> [_ w1122]
              tunnel: w1079 -> [_ w1121]
              tunnel: w1078 -> [_ w1120]
              frame #0 {
              }
              frame #1 {
                # "Write next amp.\n(wait until beginning of next loop iteration to update)"
                n207 = flat-sequence "Update the next F1 and F2 frequency value (the actual frequency won't change until FSK is switched).\nThen load the next amplitude value into buffer, but don't update it until the next cycle." {
                  tunnel: w1124 -> [w1127]
                  tunnel: w1123 -> [w1126]
                  tunnel: w1122 -> [w1125]
                  tunnel: w1121 -> [w1164]
                  tunnel: w1120 -> [w1163]
                  frame #0 {
                    n208 = for {
                      tunnel: w1127 -> [w1133] mode=indexing
                      tunnel: w1126 -> [w1132] mode=indexing
                      tunnel: w1125 -> [w1130]
                      i -> [w1131]
                      # "Write next freq."
                      n209 = To Unsigned Byte Integer(number=w1131) -> (unsigned 8bit integer=w1128:u8)
                      n210 = Add(x=w1130, y=w1128) -> (x+y=w1129:u8)
                      n211 = call "write to RF synth bd.vi"("Address Byte"=w1129, "BD 2 Byte"=w1132, "BD 1 Byte"=w1133) -> ()
                    }
                  }
                  frame #1 {
                    # "send udclk high"
                    n212 = xnode "FPGA I/O Node"("Connector1/DIO30"=TRUE ("Connector1/DIO15")) -> ()  [unwired: 1 in, 1 out]
                  }
                  frame #2 {
                    n213 = xnode "FPGA I/O Node"("Connector1/DIO30"=FALSE ("Connector1/DIO15")) -> ()  [unwired: 1 in, 1 out]
                  }
                  frame #3 {
                    n214 = for {
                      tunnel: w1164 -> [w1170] mode=indexing
                      tunnel: w1163 -> [w1169] mode=indexing
                      tunnel: u8 33 -> [w1167]
                      i -> [w1168]
                      n215 = To Unsigned Byte Integer(number=w1168) -> (unsigned 8bit integer=w1165:u8)
                      n216 = Add(x=w1167, y=w1165) -> (x+y=w1166:u8)
                      n217 = call "write to RF synth bd.vi"("Address Byte"=w1166, "BD 2 Byte"=w1169, "BD 1 Byte"=w1170) -> ()
                    }
                  }
                }
              }
            }
          }
        }
      }
    }
  }
  n218 = while "MCL stage control" {
    shift-right: [w1281] -> _
    shift-left: w1 -> [w1284]
    shift-right: [w1274] -> _
    shift-left: w5 -> [w1271]
    shift-right: [w1273] -> _
    shift-left: w4 -> [w1269]
    i -> [w1268]
    stop <- FALSE stop-if-true
    n219 = flat-sequence {
      tunnel: w1284 -> [w1288]
      tunnel: [w1289] -> w1280
      tunnel: [w1288] -> w1278
      tunnel: [w1287] -> w1272
      tunnel: w1271 -> [w1287]
      tunnel: [w1286] -> w1270
      tunnel: w1269 -> [w1286]
      tunnel: w1280 -> [w1293]
      tunnel: [w1293] -> w1279
      tunnel: w1278 -> [w1292]
      tunnel: [w1292] -> w1277
      tunnel: w1272 -> [w1291]
      tunnel: w1270 -> [w1290]
      tunnel: [w1291] -> w1267
      tunnel: [w1290] -> w1266
      tunnel: w1279 -> [w1327]
      tunnel: w1277 -> [w1326]
      tunnel: [w1327] -> w1283
      tunnel: [w1326] -> w1282
      tunnel: [w1325] -> w1276
      tunnel: [w1324] -> w1275
      tunnel: w1267 -> [w1319]
      tunnel: w1266 -> [w1318]
      tunnel: [w1391] -> w1281
      tunnel: w1283 -> [w1405]
      tunnel: w1282 -> [w1402]
      tunnel: w1276 -> [w1394]
      tunnel: w1275 -> [w1393]
      tunnel: [w1394] -> w1274
      tunnel: [w1393] -> w1273
      frame #0 {
        n220 = call "Loop Timer5"("Count(Ticks)"=w1288) -> ("Tick Count(Ticks)"=w1289:u32)
      }
      frame #1 {
        n221 = xnode "FPGA I/O Node"("Connector0/AO1"=w1291, "Connector0/AO2"=w1290) -> ()  [unwired: 2 in, 2 out]
      }
      frame #2 {
        n222 = local read "Scanning MCL"() -> (w1339:bool)
        n223 = Or(x=w1339, y="Start scan (MCL)") -> (x .or. y?=w1334:bool)
        n224 = Not(x="Abort scan (MCL)") -> (.not. x?=w1332:bool)
        n225 = And(x=w1332, y=w1334) -> (x .and. y?=w1331:bool)
        n226 = case "Raster scan" shown="True" w1331 {
          tunnel: [w1340 w1383] -> w1336
          tunnel: "Start scan (MCL)" -> [_ w1368]
          tunnel: [w1340 w1344] -> w1320
          frame #0 {
            w1340 = i16 0
            n227 = local write "Scanning MCL"(FALSE ("scanning")) -> ()
          }
          frame #1 {
            w1354 = i16 0
            w1353 = u64 0
            # "scan incr."
            # "freq. incr. mult."
            # "count steps"
            # "count number of cycles"
            n228 = feedback #16(w1353) -> (w1380:u64)
            n229 = Select(t=w1353, s=w1368, f=w1380) -> (s? t:f=w1382:u64)
            n230 = Increment(x=w1382) -> (x+1=w1379:u64)
            n231 = Greater?(x="Cycles per step (MCL)", y=w1379) -> (0:w1363:bool)
            n232 = Select(t=w1379, s=w1363, f=w1353) -> (s? t:f=w1378:u64)
            n233 = feedback #17(w1353) -> (w1377:u64)
            n234 = Select(t=w1353, s=w1368, f=w1377) -> (s? t:f=w1372:u64)
            n235 = Increment(x=w1372) -> (x+1=w1376:u64)
            n236 = Add(x="Scan steps (MCL)", y="Scan steps (MCL)") -> (x+y=w1375:u64)
            n237 = Select(t=w1372, s=w1363, f=w1376) -> (s? t:f=w1358:u64)
            n238 = Greater?(x=w1375, y=w1358) -> (0:w1357:bool)
            n239 = Select(t=w1358, s=w1357, f=w1353) -> (s? t:f=w1373:u64)
            n240 = Equal?(x="Scan steps (MCL)", y=w1358) -> (x = y?=w1362:bool)
            n241 = Greater?(x="Scan steps (MCL)", y=w1372) -> (0:w1371:bool)
            n242 = feedback #18(w1354) -> (w1374:i16)
            n243 = Select(t=w1354, s=w1368, f=w1374) -> (s? t:f=w1360:i16)
            n244 = Increment(x=w1360) -> (x+1=w1370:i16)
            n245 = Decrement(x=w1360) -> (x-1=w1369:i16)
            n246 = Select(t=w1370, s=w1371, f=w1369) -> (s? t:f=w1361:i16)
            n247 = Select(t=w1360, s=w1362, f=w1361) -> (s? t:f=w1359:i16)
            n248 = Select(t=w1360, s=w1363, f=w1359) -> (s? t:f=w1355:i16)
            n249 = Select(t=w1355, s=w1357, f=w1354) -> (s? t:f=w1356:i16)
            n250 = feedback #19(w1353) -> (w1367:u64)
            n251 = Select(t=w1353, s=w1368, f=w1367) -> (s? t:f=w1342:u64)
            n252 = Increment(x=w1342) -> (x+1=w1364:u64)
            n253 = Select(t=w1342, s=w1357, f=w1364) -> (s? t:f=w1343:u64)
            n254 = Greater?(x="Number of scans (MCL)", y=w1343) -> (0:w1350:bool)
            n255 = Multiply(x="Scan freq.  increment (MCL)", y=w1360) -> (x*y=w1383:i16)
            n256 = Select(t=TRUE, s="Cont. Scan (MCL)", f=w1350) -> (s? t:f=w1349:bool)
            "Scanning MCL" <- w1349
            n257 = Select(t=w1343, s=w1349, f=w1353) -> (s? t:f=w1365:u64)
            n258 = Increment(x=w1343) -> (x+1=→"Scan I (MCL)":u64)
            n259 = To Word Integer(number=w1342) -> (16bit integer=w1345:i16)
            n260 = Multiply(x=w1345, y="Scan freq.  increment (MCL)") -> (x*y=w1344:i16)
          }
        }
        n261 = Select(t=w1320, s="1D or 2D Scan?", f=i16 0) -> (s? t:f=w1321:i16)
        n262 = Select(t=w1321, s="MCL Scan Axis", f=w1336) -> (s? t:f=w1335:i16)
        n263 = Select(t=w1336, s="MCL Scan Axis", f=w1321) -> (s? t:f=w1337:i16)
        n264 = Add(x=w1335, y="AO2") -> (x+y=w1324:i16)
        n265 = Add(x="AO1", y=w1337) -> (x+y=w1325:i16)
        "AO1 2" <- w1319
        "AO2 2" <- w1318
      }
      frame #3 {
        n266 = feedback #20(w1405) -> (w1404:u32)
        n267 = Boolean To (0,1)(Boolean="+ phase (MCL)") -> (0, 1=w1389:i16)
        n268 = Subtract(x=w1405, y=w1404) -> (x-y=w1403:u32)
        n269 = Multiply(x=w1389, y="Phase count adjustment (MCL)") -> (x*y=w1385:i16)
        n270 = Subtract(x=w1403, y=w1402) -> (x-y=w1400:u32)
        n271 = Subtract(x="MCL count", y=w1400) -> (x-y=w1387:u32)
        n272 = feedback #21(i16 0) -> (w1386:i16)
        n273 = Subtract(x=w1386, y=w1385) -> (x-y=w1384:i16)
        "MCL Relative Phase" <- w1384
        n274 = Greater?(x=w1400, y=u32 0) -> (0:w1399:bool)
        "MCL Late?" <- w1399
        n275 = Add(x=w1387, y=w1385) -> (x+y=w1391:u32)
        n276 = feedback #22(u32 0) -> (w1397:u32)
        n277 = Increment(x=w1397) -> (x+1=w1396:u32)
        n278 = Select(t=w1396, s=w1399, f=w1397) -> (s? t:f=w1398:u32)
        "MCL Late Counter" <- w1398
      }
    }
    "Numeric" <- w1268
  }
  n279 = while "APD Gating" {
    shift-right: [w1410] -> _
    shift-left: w1 -> [w1415]
    shift-right: [w1409] -> _
    shift-left: FALSE -> [w1407]
    stop <- FALSE stop-if-true
    n280 = flat-sequence {
      tunnel: w1415 -> [w1418]
      tunnel: [w1419] -> w1413
      tunnel: [w1418] -> w1411
      tunnel: [w1417] -> w1408
      tunnel: w1407 -> [w1417]
      tunnel: [w1422] -> w1414
      tunnel: w1413 -> [w1422]
      tunnel: [w1421] -> w1412
      tunnel: w1411 -> [w1421]
      tunnel: w1408 -> [w1420]
      tunnel: [w1516] -> w1410
      tunnel: w1414 -> [w1538]
      tunnel: w1412 -> [w1535]
      tunnel: [w1521] -> w1409
      frame #0 {
        n281 = call "Loop Timer7"("Count(Ticks)"=w1418) -> ("Tick Count(Ticks)"=w1419:u32)
      }
      frame #1 {
        # "Can switch 2 APDs\n(need 4 channels/APD)"
        n282 = xnode "FPGA I/O Node"("Connector0/DIO4"=w1420, "Connector0/DIO5"=w1420, "Connector0/DIO6"=w1420, "Connector0/DIO7"=w1420, "Connector0/DIO8"=w1420, "Connector0/DIO9"=w1420, "Connector0/DIO10"=w1420, "Connector0/DIO11"=w1420) -> ()  [unwired: 8 in, 8 out]
      }
      frame #2 {
        n283 = feedback #23(TRUE) -> (w1524:bool)
        n284 = feedback #24(w1538) -> (w1537:u32)
        n285 = Not(x=w1524) -> (.not. x?=w1520:bool)
        n286 = Subtract(x=w1538, y=w1537) -> (x-y=w1536:u32)
        n287 = Select(t="APD Gate ON Count", s=w1520, f="APD Gate OFF Count") -> (s? t:f=w1526:u32)
        n288 = Subtract(x=w1536, y=w1535) -> (x-y=w1527:u32)
        n289 = Subtract(x=w1526, y=w1527) -> (x-y=w1515:u32)
        n290 = Greater?(x=w1527, y=u32 0) -> (0:w1531:bool)
        "APD Gate Late?" <- w1531
        n291 = Boolean To (0,1)(Boolean="+ phase (APD Gate)") -> (0, 1=w1513:i16)
        n292 = Multiply(x=w1513, y="Phase count adjustment (APD Gate)") -> (x*y=w1511:i16)
        n293 = feedback #25(u32 0) -> (w1533:u32)
        n294 = Increment(x=w1533) -> (x+1=w1532:u32)
        n295 = Select(t=w1532, s=w1531, f=w1533) -> (s? t:f=w1530:u32)
        "APD Gate Late Counter" <- w1530
        n296 = Add(x=w1515, y=w1511) -> (x+y=w1516:u32)
        n297 = feedback #26(i16 0) -> (w1518:i16)
        n298 = Subtract(x=w1518, y=w1511) -> (x-y=w1517:i16)
        "APD Gate Relative Phase" <- w1517
        n299 = case shown="2" "APD Gate Operating Mode" {
          tunnel: [TRUE FALSE w1544] -> w1521
          tunnel: w1524 -> [_ _ w1541]
          frame #0 {
          }
          frame #1 {
          }
          frame #2 {
            n300 = Not(x=w1541) -> (.not. x?=w1543:bool)
            n301 = Select(t=w1543, s="Invert APD Gate", f=w1541) -> (s? t:f=w1544:bool)
          }
        }
      }
    }
  }
  n302 = while "RF box board direct communication loop" {
    tunnel: w1 -> [_]
    stop <- FALSE stop-if-true
    n303 = case "Whether to use direct communication method (only use one method at a time)" shown="True" "Direct RF Box \nCommunication" {
      frame #0 {
      }
      frame #1 {
        n304 = case shown="True" "Update Data" {
          frame #0 {
          }
          frame #1 {
            n305 = flat-sequence {
              frame #0 {
                n306 = First Call?() -> (First Call?: T/F=w1548:bool)
                n307 = case shown="True" w1548 {
                  frame #0 {
                  }
                  frame #1 {
                    # "If first time data updated, be sure to set WR high\nbefore setting data and address bits."
                    n308 = flat-sequence {
                      frame #0 {
                        n309 = xnode "FPGA I/O Node"("Connector1/DIO15"=TRUE) -> ()  [unwired: 1 in, 1 out]
                      }
                      frame #1 {
                        n310 = call "Wait"("Count(Ticks)"=u8 40 ("DO Delay 3 (Ticks)")) -> ()  [unwired: 1 out]
                      }
                    }
                  }
                }
              }
              frame #1 {
                n311 = Number To Boolean Array(number="Address") -> (Boolean array=w1610:bool[])
                n312 = Number To Boolean Array(number="Data BD 1") -> (Boolean array=w1611:bool[])
                n313 = Number To Boolean Array(number="Data BD 2") -> (Boolean array=w1580:bool[])
                n314 = Index Array(array=w1611, index=7) -> (element=w1595:bool)
                n315 = Index Array(array=w1611, index=6) -> (element=w1594:bool)
                n316 = Index Array(array=w1611, index=5) -> (element=w1593:bool)
                n317 = Index Array(array=w1611, index=4) -> (element=w1592:bool)
                n318 = Index Array(array=w1611, index=3) -> (element=w1591:bool)
                n319 = Index Array(array=w1611, index=2) -> (element=w1590:bool)
                n320 = Index Array(array=w1611, index=1) -> (element=w1589:bool)
                n321 = Index Array(array=w1611, index=0) -> (element=w1588:bool)
                n322 = Index Array(array=w1610, index=5) -> (element=w1587:bool)
                n323 = Index Array(array=w1610, index=4) -> (element=w1586:bool)
                n324 = Index Array(array=w1610, index=3) -> (element=w1585:bool)
                n325 = Index Array(array=w1610, index=2) -> (element=w1584:bool)
                n326 = Index Array(array=w1610, index=1) -> (element=w1583:bool)
                n327 = Index Array(array=w1610, index=0) -> (element=w1582:bool)
                n328 = Index Array(array=w1580, index=7) -> (element=w1571:bool)
                n329 = Index Array(array=w1580, index=6) -> (element=w1570:bool)
                n330 = Index Array(array=w1580, index=5) -> (element=w1569:bool)
                n331 = Index Array(array=w1580, index=4) -> (element=w1568:bool)
                n332 = Index Array(array=w1580, index=3) -> (element=w1567:bool)
                n333 = Index Array(array=w1580, index=2) -> (element=w1566:bool)
                n334 = Index Array(array=w1580, index=1) -> (element=w1565:bool)
                n335 = Index Array(array=w1580, index=0) -> (element=w1564:bool)
                n336 = xnode "FPGA I/O Node"("Connector1/DIO0"=w1595, "Connector1/DIO1"=w1594, "Connector1/DIO2"=w1593, "Connector1/DIO3"=w1592, "Connector1/DIO4"=w1591, "Connector1/DIO5"=w1590, "Connector1/DIO6"=w1589, "Connector1/DIO7"=w1588, "Connector1/DIO8"=w1587, "Connector1/DIO9"=w1586, "Connector1/DIO10"=w1585, "Connector1/DIO11"=w1584, "Connector1/DIO12"=w1583, "Connector1/DIO13"=w1582, "Connector1/DIO20"=w1571, "Connector1/DIO21"=w1570, "Connector1/DIO22"=w1569, "Connector1/DIO23"=w1568, "Connector1/DIO24"=w1567, "Connector1/DIO25"=w1566, "Connector1/DIO26"=w1565, "Connector1/DIO27"=w1564) -> ()  [unwired: 22 in, 22 out]
              }
              frame #2 {
                # "wait and then apply write signal"
                n337 = call "Wait2"("Count(Ticks)"=u8 40 ("DO Delay 1 (Ticks)")) -> ()  [unwired: 1 out]
              }
              frame #3 {
                # "sending bit low writes data to board buffer"
                n338 = xnode "FPGA I/O Node"("Connector1/DIO15"=FALSE) -> ()  [unwired: 1 in, 1 out]
              }
              frame #4 {
                # "wait then return write signal"
                n339 = call "Wait3"("Count(Ticks)"=u8 40 ("DO Delay 2 (Ticks)")) -> ()  [unwired: 1 out]
              }
              frame #5 {
                # "sending bit high makes ready to\nwrite more data"
                n340 = xnode "FPGA I/O Node"("Connector1/DIO15"=TRUE) -> ()  [unwired: 1 in, 1 out]
              }
            }
          }
        }
      }
    }
  }
  n341 = while "Control Additional IO (Green laser flip mount)" {
    stop <- FALSE stop-if-true
    n342 = xnode "FPGA I/O Node"("Connector0/DIO3"="Green Filter Flipper", "Connector0/DIO2"="Connector0/DIO9", "Connector1/DIO32"="Connector1/DIO32", "Connector1/DIO33"="Connector1/DIO33", "Connector1/DIO34"="Connector1/DIO34", "Chassis2/Mod4/AO1"="Chassis2/Mod4/AO1") -> ()  [unwired: 6 in, 6 out]
    n343 = call "Loop Timer2"("Count(Ticks)"="Extra DO Counts") -> ()  [unwired: 1 out]
  }
  n344 = while "Control APD data integration - stream to host" {
    shift-right: [w2006] -> _
    shift-left: w1 -> [w2011]
    stop <- FALSE stop-if-true
    n345 = flat-sequence {
      tunnel: w2011 -> [w2013]
      tunnel: [w2014] -> w2009
      tunnel: [w2013] -> w2007
      tunnel: [w2022] -> w2010
      tunnel: w2009 -> [w2022]
      tunnel: [w2021] -> w2008
      tunnel: w2007 -> [w2021]
      tunnel: [w2020] -> w2005
      tunnel: [w2019] -> w2004
      tunnel: [w2046] -> w2006
      tunnel: w2010 -> [w2071]
      tunnel: w2008 -> [w2068]
      tunnel: w2005 -> [w2039]
      tunnel: w2004 -> [w2038]
      frame #0 {
        n346 = call "Loop Timer6"("Count(Ticks)"=w2013) -> ("Tick Count(Ticks)"=w2014:u32)
      }
      frame #1 {
        n347 = flat-sequence {
          tunnel: [w2023] -> w2018
          tunnel: w2018 -> [w2026]
          tunnel: [w2028] -> w2017
          tunnel: [w2027] -> w2016
          tunnel: [w2026] -> w2015
          tunnel: [w2034] -> w2019
          tunnel: [w2035] -> w2020
          tunnel: w2017 -> [w2035]
          tunnel: w2016 -> [w2034]
          tunnel: w2015 -> [w2033]
          frame #0 {
            n348 = feedback #27(FALSE) -> (w2024:bool)
            "APD out state" <- w2024
            n349 = Not(x=w2024) -> (.not. x?=w2023:bool)
          }
          frame #1 {
            n350 = local read "APD 1 Counts 1"() -> (w2032:u32)
            n351 = local read "APD 1 Counts 0"() -> (w2031:u32)
            n352 = local read "APD 2 Counts 1"() -> (w2030:u32)
            n353 = local read "APD 2 Counts 0"() -> (w2029:u32)
            n354 = Select(t=w2032, s=w2026, f=w2031) -> (s? t:f=w2028:u32)
            n355 = Select(t=w2030, s=w2026, f=w2029) -> (s? t:f=w2027:u32)
          }
          frame #2 {
            n356 = case shown="False" w2033 {
              frame #0 {
                w2036 = u32 0 ("APD 1 Counts 0")
                n357 = local write "APD 1 Counts 0"(w2036) -> ()
                n358 = local write "APD 2 Counts 0"(w2036) -> ()
              }
              frame #1 {
                w2037 = u32 0 ("APD 1 Counts 1")
                n359 = local write "APD 1 Counts 1"(w2037) -> ()
                n360 = local write "APD 2 Counts 1"(w2037) -> ()
              }
            }
          }
        }
      }
      frame #2 {
        n361 = feedback #28(w2071) -> (w2070:u32)
        n362 = Subtract(x=w2071, y=w2070) -> (x-y=w2069:u32)
        n363 = Subtract(x=w2069, y=w2068) -> (x-y=w2062:u32)
        n364 = case shown="True" "APD to FIFO" {
          tunnel: w2039 -> [_ w2098]
          tunnel: w2038 -> [_ w2096]
          frame #0 {
          }
          frame #1 {
            n365 = flat-sequence {
              tunnel: 0 ("Timeout") -> [w2100]
              tunnel: w2098 -> [w2101]
              tunnel: [w2100] -> w2097
              tunnel: w2097 -> [w2128]
              tunnel: w2096 -> [w2127]
              frame #0 {
                n366 = xnode ("FIFO Write")("Element"=w2101, "Timeout"=w2100) -> ()  [unwired: 1 in, 2 out]
              }
              frame #1 {
                n367 = xnode ("FIFO Write")("Element"=w2127, "Timeout"=w2128) -> ()  [unwired: 1 in, 2 out]
              }
            }
          }
        }
        n368 = Subtract(x="APD Acq Rate Count", y=w2062) -> (x-y=w2047:u32)
        n369 = Greater?(x=w2062, y=u32 0) -> (0:w2064:bool)
        "APD Acq Late?" <- w2064
        n370 = feedback #29(u32 0) -> (w2066:u32)
        n371 = Increment(x=w2066) -> (x+1=w2065:u32)
        n372 = Select(t=w2065, s=w2064, f=w2066) -> (s? t:f=w2063:u32)
        "APD Acq Late Counter" <- w2063
        n373 = Boolean To (0,1)(Boolean="+ phase (APD Acq)") -> (0, 1=w2043:i16)
        n374 = Multiply(x=w2043, y="Phase Count Adjustment (APD Acq)") -> (x*y=w2040:i16)
        n375 = Add(x=w2047, y=w2040) -> (x+y=w2046:u32)
        n376 = feedback #30(i16 0) -> (w2045:i16)
        n377 = Subtract(x=w2045, y=w2040) -> (x-y=w2042:i16)
        "APD Acq Relative Phase" <- w2042
        n378 = To Word Integer(number=w2039) -> (16bit integer=w2055:i16)
        n379 = To Word Integer(number=w2038) -> (16bit integer=w2056:i16)
        n380 = Multiply(x="APD 1 AO scale factor", y=w2055) -> (x*y=w2054:i16)
        n381 = Multiply(x="APD 2 AO scale factor", y=w2056) -> (x*y=w2053:i16)
        n382 = Add(x="APD 1 AO offset", y=w2054) -> (x+y=w2052:i16)
        n383 = Add(x=w2053, y="APD 2 AO offset") -> (x+y=w2050:i16)
        n384 = xnode "FPGA I/O Node"("Connector0/AO6"=w2052, "Connector0/AO7"=w2050) -> ()  [unwired: 2 in, 2 out]
      }
    }
  }
  n385 = timed-loop "RF box board DIO control: control bits" {
    timing: w3 -> [_]
    timing-out: [_] -> w2
    tunnel: [w2154] -> _
    tunnel: w1 -> [w2154]
    stop <- FALSE stop-if-true
    n386 = xnode "FPGA I/O Node"("Connector1/DIO16"="RD", "Connector1/DIO17"="PMODE", "Connector1/DIO18"="OSK Bd 1", "Connector1/DIO19"="Reset Bd 1", "Connector1/DIO28"="OSK Bd 2", "Connector1/DIO29"="Reset Bd 2") -> ()  [unwired: 6 in, 6 out]
  }
  n387 = while "Green excitation laser feedback measurement" {
    shift-right: [w2242] -> _
    shift-left: w1 -> [w2247]
    stop <- FALSE stop-if-true
    n388 = flat-sequence {
      tunnel: w2247 -> [w2249]
      tunnel: [w2250] -> w2245
      tunnel: [w2249] -> w2243
      tunnel: [w2257] -> w2246
      tunnel: w2245 -> [w2257]
      tunnel: [w2256] -> w2244
      tunnel: w2243 -> [w2256]
      tunnel: [w2333] -> w2242
      tunnel: w2246 -> [w2351]
      tunnel: w2244 -> [w2348]
      frame #0 {
        n389 = call "Loop Timer9"("Count(Ticks)"=w2249) -> ("Tick Count(Ticks)"=w2250:u32)
      }
      frame #1 {
        n390 = xnode "FPGA I/O Node"("Connector1/DIO35"=TRUE) -> ("Chassis2/Mod1/AI0"=w2255:i16, "Chassis2/Mod1/AI1"=w2254:i16, "Chassis2/Mod1/AI2"=w2251:i16)  [unwired: 4 in, 4 out]
        "Green FB Sum" <- w2251
        n391 = Bundle("Chassis2/Mod1/AI0"=w2255, "Chassis2/Mod1/AI1"=w2254, "Chassis2/Mod1/AI2"=w2251) -> (→"Green FB Signals":T12)  [unwired: 1 out]
      }
      frame #2 {
        n392 = feedback #31(w2351) -> (w2350:u32)
        n393 = Subtract(x=w2351, y=w2350) -> (x-y=w2349:u32)
        n394 = xnode "FPGA I/O Node"("Connector1/DIO35"=FALSE) -> ()  [unwired: 1 in, 1 out]
        n395 = Subtract(x=w2349, y=w2348) -> (x-y=w2342:u32)
        n396 = Subtract(x="Green FB Count", y=w2342) -> (x-y=w2337:u32)
        n397 = Greater?(x=w2342, y=u32 0) -> (0:w2344:bool)
        "Green FB Late?" <- w2344
        n398 = Boolean To (0,1)(Boolean="+ phase (Green FB)") -> (0, 1=w2335:i16)
        n399 = Multiply(x=w2335, y="Phase count adjustment (Green FB)") -> (x*y=w2330:i16)
        n400 = feedback #32(u32 0) -> (w2346:u32)
        n401 = Increment(x=w2346) -> (x+1=w2345:u32)
        n402 = Select(t=w2345, s=w2344, f=w2346) -> (s? t:f=w2343:u32)
        "Green Late Counter" <- w2343
        n403 = Add(x=w2337, y=w2330) -> (x+y=w2333:u32)
        n404 = feedback #33(i16 0) -> (w2332:i16)
        n405 = Subtract(x=w2332, y=w2330) -> (x-y=w2331:i16)
        "Green FB Relative Phase" <- w2331
      }
    }
  }
  n406 = while "Green fluorescent laser interlacing (DO to IA 532 nm AOM ME amp)." {
    shift-right: [w2367] -> _
    shift-left: w1 -> [w2372]
    shift-right: [w2366] -> _
    shift-left: FALSE -> [w2364]
    stop <- FALSE stop-if-true
    n407 = flat-sequence {
      tunnel: w2372 -> [w2375]
      tunnel: [w2376] -> w2370
      tunnel: [w2375] -> w2368
      tunnel: [w2374] -> w2365
      tunnel: w2364 -> [w2374]
      tunnel: [w2379] -> w2371
      tunnel: w2370 -> [w2379]
      tunnel: [w2378] -> w2369
      tunnel: w2368 -> [w2378]
      tunnel: w2365 -> [w2377]
      tunnel: [w2419] -> w2367
      tunnel: w2371 -> [w2446]
      tunnel: w2369 -> [w2443]
      tunnel: [w2429] -> w2366
      frame #0 {
        n408 = call "Loop Timer4"("Count(Ticks)"=w2375) -> ("Tick Count(Ticks)"=w2376:u32)
      }
      frame #1 {
        n409 = xnode "FPGA I/O Node"("Connector1/DIO37"=w2377, "Connector1/DIO38"=w2377, "Connector1/DIO39"=w2377) -> ()  [unwired: 3 in, 3 out]
      }
      frame #2 {
        n410 = feedback #34(w2446) -> (w2445:u32)
        n411 = Subtract(x=w2446, y=w2445) -> (x-y=w2444:u32)
        n412 = Subtract(x=w2444, y=w2443) -> (x-y=w2435:u32)
        n413 = Greater?(x=w2435, y=u32 0) -> (0:w2439:bool)
        "GI Late?" <- w2439
        n414 = Boolean To (0,1)(Boolean="+ phase (GI)") -> (0, 1=w2424:i16)
        n415 = Multiply(x=w2424, y="Phase count adjustment (GI)") -> (x*y=w2421:i16)
        n416 = feedback #35(u32 0) -> (w2441:u32)
        n417 = Increment(x=w2441) -> (x+1=w2440:u32)
        n418 = Select(t=w2440, s=w2439, f=w2441) -> (s? t:f=w2438:u32)
        "GI Late Counter" <- w2438
        n419 = feedback #36(i16 0) -> (w2422:i16)
        n420 = Subtract(x=w2422, y=w2421) -> (x-y=w2420:i16)
        "GI Relative phase" <- w2420
        n421 = feedback #37(TRUE) -> (w2432:bool)
        n422 = case shown="2" "Operating Mode" {
          tunnel: [TRUE FALSE w2452] -> w2429
          tunnel: w2432 -> [_ _ w2449]
          frame #0 {
          }
          frame #1 {
          }
          frame #2 {
            n423 = Not(x=w2449) -> (.not. x?=w2451:bool)
            n424 = Select(t=w2451, s="Invert GI", f=w2449) -> (s? t:f=w2452:bool)
          }
        }
        n425 = Not(x=w2432) -> (.not. x?=w2428:bool)
        n426 = Select(t="Green interlace ON count", s=w2428, f="Green interlace OFF count") -> (s? t:f=w2434:u32)
        n427 = Subtract(x=w2434, y=w2435) -> (x-y=w2425:u32)
        n428 = Add(x=w2425, y=w2421) -> (x+y=w2419:u32)
      }
    }
  }
  n429 = while "Green fluorescent laser interlacing (Current to IA 532 nm AOM ME amp)." {
    shift-right: [w2458] -> _
    shift-left: w1 -> [w2461]
    shift-right: [w2455] -> _
    shift-left: w1 -> [w2453]
    stop <- FALSE stop-if-true
    n430 = flat-sequence {
      tunnel: w2461 -> [w2464]
      tunnel: [w2465] -> w2460
      tunnel: [w2464] -> w2459
      tunnel: [w2463] -> w2454
      tunnel: w2453 -> [w2463]
      tunnel: [w2468] -> w2457
      tunnel: w2460 -> [w2468]
      tunnel: [w2467] -> w2456
      tunnel: w2459 -> [w2467]
      tunnel: w2454 -> [w2466]
      tunnel: [w2481] -> w2458
      tunnel: [w2499] -> w2455
      tunnel: w2457 -> [w2518]
      tunnel: w2456 -> [w2515]
      frame #0 {
        n431 = call "Loop Timer10"("Count(Ticks)"=w2464) -> ("Tick Count(Ticks)"=w2465:u32)
      }
      frame #1 {
        n432 = xnode "FPGA I/O Node"("Chassis2/Mod4/AO0"=w2466) -> ()  [unwired: 1 in, 1 out]
      }
      frame #2 {
        n433 = Subtract(x="Green interlace OFF count 2", y="Green int current ON count adj") -> (x-y=w2491:u32)
        n434 = feedback #38(w2518) -> (w2517:u32)
        n435 = Add(x="Green int current ON count adj", y="Green interlace ON count 2") -> (x+y=w2492:u32)
        n436 = Subtract(x=w2518, y=w2517) -> (x-y=w2516:u32)
        n437 = Subtract(x=w2516, y=w2515) -> (x-y=w2507:u32)
        n438 = Greater?(x=w2507, y=u32 0) -> (0:w2511:bool)
        "GI Late? 2" <- w2511
        n439 = Boolean To (0,1)(Boolean="+ phase (GI) 2") -> (0, 1=w2487:i16)
        n440 = Multiply(x=w2487, y="Phase count adjustment (GI) 2") -> (x*y=w2483:i16)
        n441 = feedback #39(u32 0) -> (w2513:u32)
        n442 = Increment(x=w2513) -> (x+1=w2512:u32)
        n443 = Select(t=w2512, s=w2511, f=w2513) -> (s? t:f=w2510:u32)
        "GI Late Counter 2" <- w2510
        n444 = feedback #40(i16 0) -> (w2484:i16)
        n445 = Subtract(x=w2484, y=w2483) -> (x-y=w2482:i16)
        "GI Relative phase 2" <- w2482
        n446 = feedback #41(TRUE) -> (w2504:bool)
        n447 = case shown="2" "Operating Mode 2" {
          tunnel: [TRUE FALSE w2535] -> w2493
          tunnel: w2504 -> [_ _ w2532]
          frame #0 {
          }
          frame #1 {
          }
          frame #2 {
            n448 = Not(x=w2532) -> (.not. x?=w2534:bool)
            n449 = Select(t=w2534, s="Invert GI 2", f=w2532) -> (s? t:f=w2535:bool)
          }
        }
        n450 = And(x=w2493, y="Green FB On/Off") -> (x .and. y?=w2494:bool)
        n451 = case shown="True" w2494 {
          tunnel: "Current Out" -> [w2519 _]
          tunnel: [w2519 w2524] -> w2498
          frame #0 {
          }
          frame #1 {
            n452 = local read "Green FB Sum"() -> (w2520:i16)
            n453 = call "Slower PID.vi"("process variable"=w2520, "reset?"="Green FB Reset", "setpoint"="Green FB Setpoint", "PID gains (x 2^8)"="Green FB Gains", "output range"=cluster{"output high":i16, "output low":i16} {"output high"=32767, "output low"=-32768} ("Green FB output range")) -> ("output"=w2528:i16)  [unwired: 10 out]
            n454 = To Long Integer(number=w2528) -> (32bit integer=w2521:i32)
            n455 = Add(x=w2521, y=32768) -> (x+y=w2523:i32)
            n456 = To Unsigned Word Integer(number=w2523) -> (unsigned 16bit integer=w2524:u16)
          }
        }
        n457 = Not(x=w2504) -> (.not. x?=w2501:bool)
        n458 = Select(t=w2492, s=w2501, f=w2491) -> (s? t:f=w2506:u32)
        n459 = Subtract(x=w2506, y=w2507) -> (x-y=w2485:u32)
        n460 = Add(x=w2485, y=w2483) -> (x+y=w2481:u32)
        n461 = Boolean To (0,1)(Boolean=w2493) -> (0, 1=w2500:i16)
        n462 = To Unsigned Word Integer(number=w2500) -> (unsigned 16bit integer=w2497:u16)
        n463 = Multiply(x=w2497, y=w2498) -> (x*y=w2499:u16)
      }
    }
  }
  n464 = node-c288(w2) -> ()
